vi "Find term type by ID (Terminal).vi"(7 "Search ID":string, 8 "error in (no error)":errorcluster, 11 "Term Types":cluster{"Terminal":refnum<vi>, "Id":string}[](array[cluster])) -> (0 "error out":errorcluster, 1 "Terminal":cluster{"Terminal":refnum<vi>, "Id":string}, 2 "index of term":i32, 3 "Other Term Types":cluster{"Terminal":refnum<vi>, "Id":string}[](array[cluster]), 5 "Found ?":bool)   [LabVIEW 2018, in "Scripting Tools.lvlib" / "XNode Support.lvlib"]
doc: "Search the <b>term types</b> array for one with the <b>Search ID</b> and return the corresponding <b>Term Type</b>. If found then returns true to <b>Found?</b>."
uses:
  XNode Support.lvlib
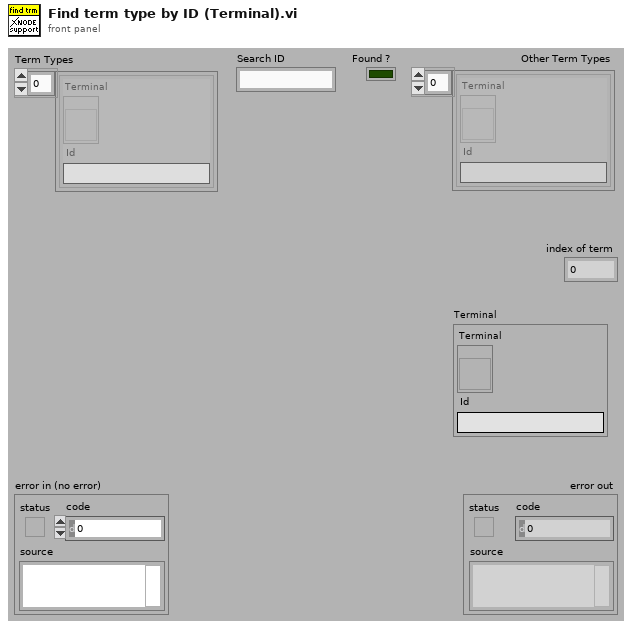
[diagram p1: front panel]
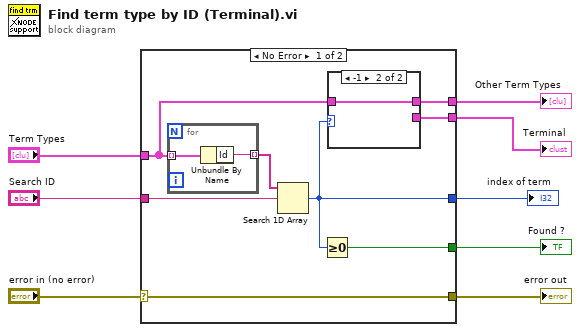
[diagram p0: block diagram]
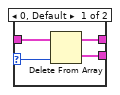
[diagram p2: hidden frame]
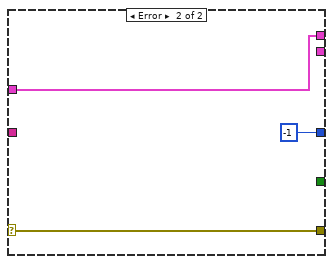
[diagram p3: hidden frame]
diagram:
  n1 = case shown="No Error" "error in (no error)" {
    selector: "error in (no error)" -> [w11 w26]
    tunnel: [w11 w26] -> w7
    tunnel: [w14 _] -> w6
    tunnel: [w12 _] -> w1
    tunnel: "Term Types" -> [w13 w24]
    tunnel: "Search ID" -> [w15 _]
    tunnel: [w9 -1 ("index of element")] -> w3
    tunnel: [w10 w24] -> w2
    frame No Error {
      n2 = for {
        tunnel: w13 -> [w23] mode=indexing
        tunnel: [w22] -> w16 mode=indexing
        n3 = Unbundle By Name(w23) -> ("Id"=w22:string)
      }
      n4 = Search 1D Array(1D array=w16, element=w15) -> (index of element=w9:i32)  [unwired: 1 out]
      n5 = Greater Or Equal To 0?(x=w9) -> (x >= 0?=w14:bool)
      n6 = case shown="-1" w9 {
        selector: w9 -> [w17 _]
        tunnel: w13 -> [w20 w21]
        tunnel: [w19 _] -> w12
        tunnel: [w18 w21] -> w10
        frame 0, Default {
          n7 = Delete From Array(array=w20, index=w17) -> (deleted portion=w19:cluster{"Terminal":refnum<vi>, "Id":string}, array with subset deleted=w18:cluster{"Terminal":refnum<vi>, "Id":string}[])  [unwired: 1 in]
        }
        frame -1 {
        }
      }
    }
    frame Error {
    }
  }
  "error out" <- w7
  "Found ?" <- w6
  "index of term" <- w3
  "Other Term Types" <- w2
  "Terminal" <- w1
